vi "Find_error_type.vi"(11 "Error In":T1) -> (15 "Error Type":string)   [LabVIEW 2020]
doc: "This VI is used to find the type of the error that is occured in the PSRR vi."
uses:
  Typedef's/Error_Cluster.ctl
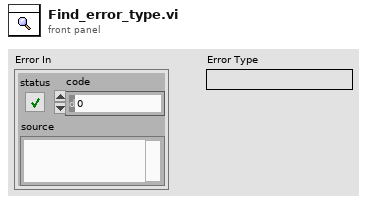
[diagram p1: front panel]
types:
  T1 = typedef "Error_Cluster.ctl" = errorcluster
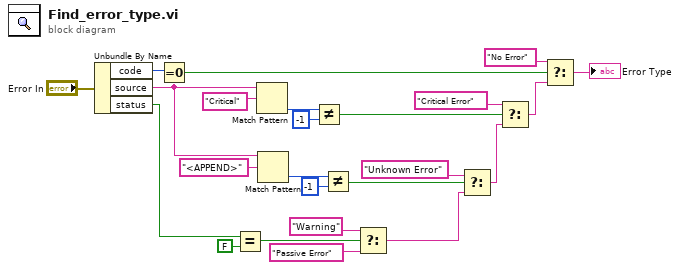
[diagram p0: block diagram]
diagram:
  n1 = Unbundle By Name("Error In") -> ("code"=w7:i32, "source"=w15:string, "status"=w18:bool)
  n2 = Equal To 0?(x=w7) -> (x = 0?=w20:bool)
  n3 = Equal?(x=w18, y=FALSE) -> (x = y?=w16:bool)
  n4 = Match Pattern(string=w15, regular expression="Critical") -> (offset past match=w23:i32)  [unwired: 1 in, 3 out]
  n5 = Match Pattern(string=w15, regular expression="<APPEND>") -> (offset past match=w12:i32)  [unwired: 1 in, 3 out]
  n6 = Not Equal?(x=w23, y=-1) -> (x != y?=w21:bool)
  n7 = Not Equal?(x=w12, y=-1) -> (x != y?=w11:bool)
  n8 = Select(t="Warning", s=w16, f="Passive Error") -> (s? t:f=w9:string)
  n9 = Select(t="Unknown Error", s=w11, f=w9) -> (s? t:f=w10:string)
  n10 = Select(t="Critical Error", s=w21, f=w10) -> (s? t:f=w19:string)
  n11 = Select(t="No Error", s=w20, f=w19) -> (s? t:f=→"Error Type":string)
